vi "StateLED.vi"(0 "Master State":T1(ring)) -> ()   [LabVIEW 2019]
doc: "This VI manages the apperance of the LEDs. The LED coloration and blink pattern report the robot mode and status. See project documentation for details."
uses:
  outputs.vi
  dscommands.vi
  refnums.vi
  dsdata.vi
  sensors.vi
  autoninfo.vi
  <vilib>/vision/NI_Vision_Development_Module.lvlib
panel:
  in  "Shooter Firing":u32(colorbox)=61212
  in  "Shooter Ready":u32(colorbox)=16711758
  in  "User Value Choice":u8(slide)=255 step=1 scale=0.0..255.0
  in  "User Saturation Choice":u8(slide)=255 step=1 scale=0.0..255.0
  in  "Pressure Insert":u32(colorbox)=91
  in  "Battery Insert":u32(colorbox)=65282
  in  "Pressure Background":u32(colorbox)=16711680
  in  "Battery Background":u32(colorbox)=16711680
  in  "Pressure LED Length":i32=5
  in  "Battery LED Length":i32=5
  in  "Battery Index":i32=1
  in  "Pressure Index":i32=15
  in  "Swerve 3 LED Index":i32=20
  in  "Swerve 2 LED Index":i32
  in  "Swerve 1 LED Index":i32=6
  in  "Swerve LED Length":i32=1
  in  "Swerve 0 LED Index":i32=14
  in  "Locate LED":bool
  in  "LED Index":i32
  out "User Blue":u8
  out "User Green":u8=255
  out "User Red":u8
  in  "Choose Hue":bool
  in  "User Hue Choice":u8(slide) step=1 scale=0.0..255.0
  in  "Nominal Chase":u32(colorbox)=65280
  in  "Spinning":u32(colorbox)=16765440
  in  "Human Player Signal (blink)":u32(colorbox)=6618880
  in  "Diverting Power":u32(colorbox)
  in  "Master Caution Chase":u32(colorbox)=16711680
  in  "Autonomous Chase":u32(colorbox)=16727040
  in  "Human Driving":u32(colorbox)=43263
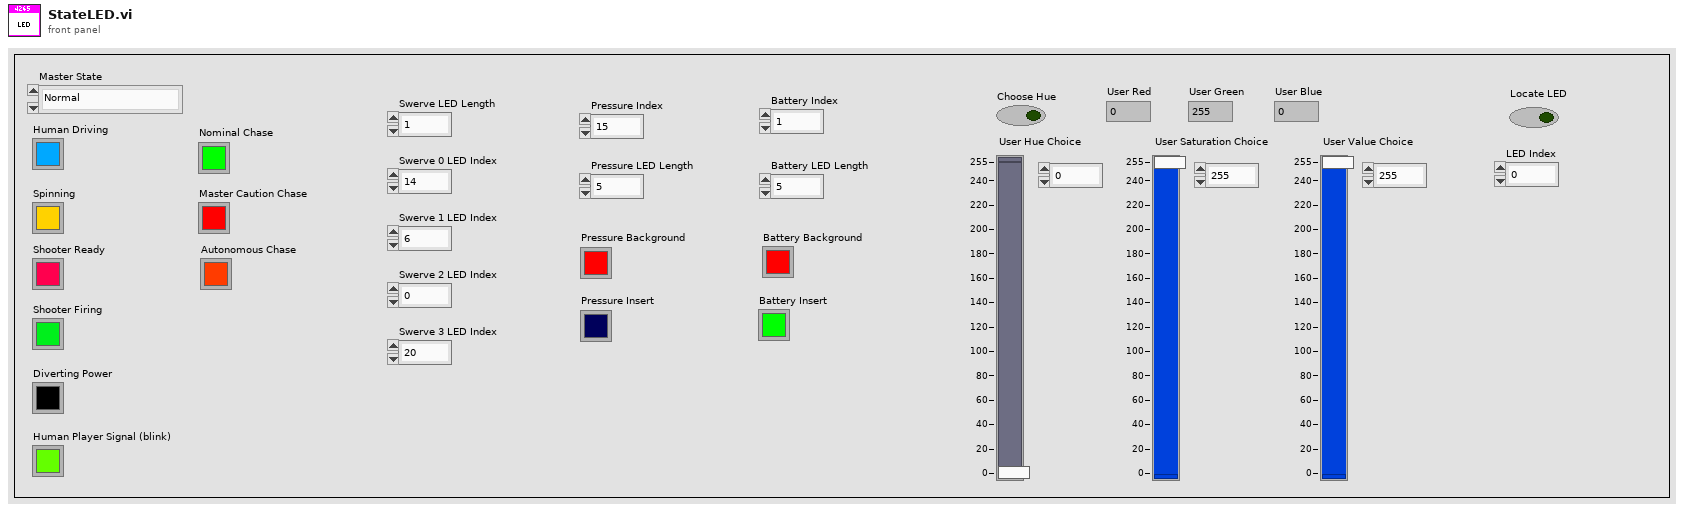
[diagram p1: front panel]
types:
  T1 = enum16{"Normal", "Control Rotation", "Control Position", "Climb"}
  T2 = enum16{"Normal", "Party Mode", "Choose Hue", "Debug", "Locate LED", "Rainbow Distance"}
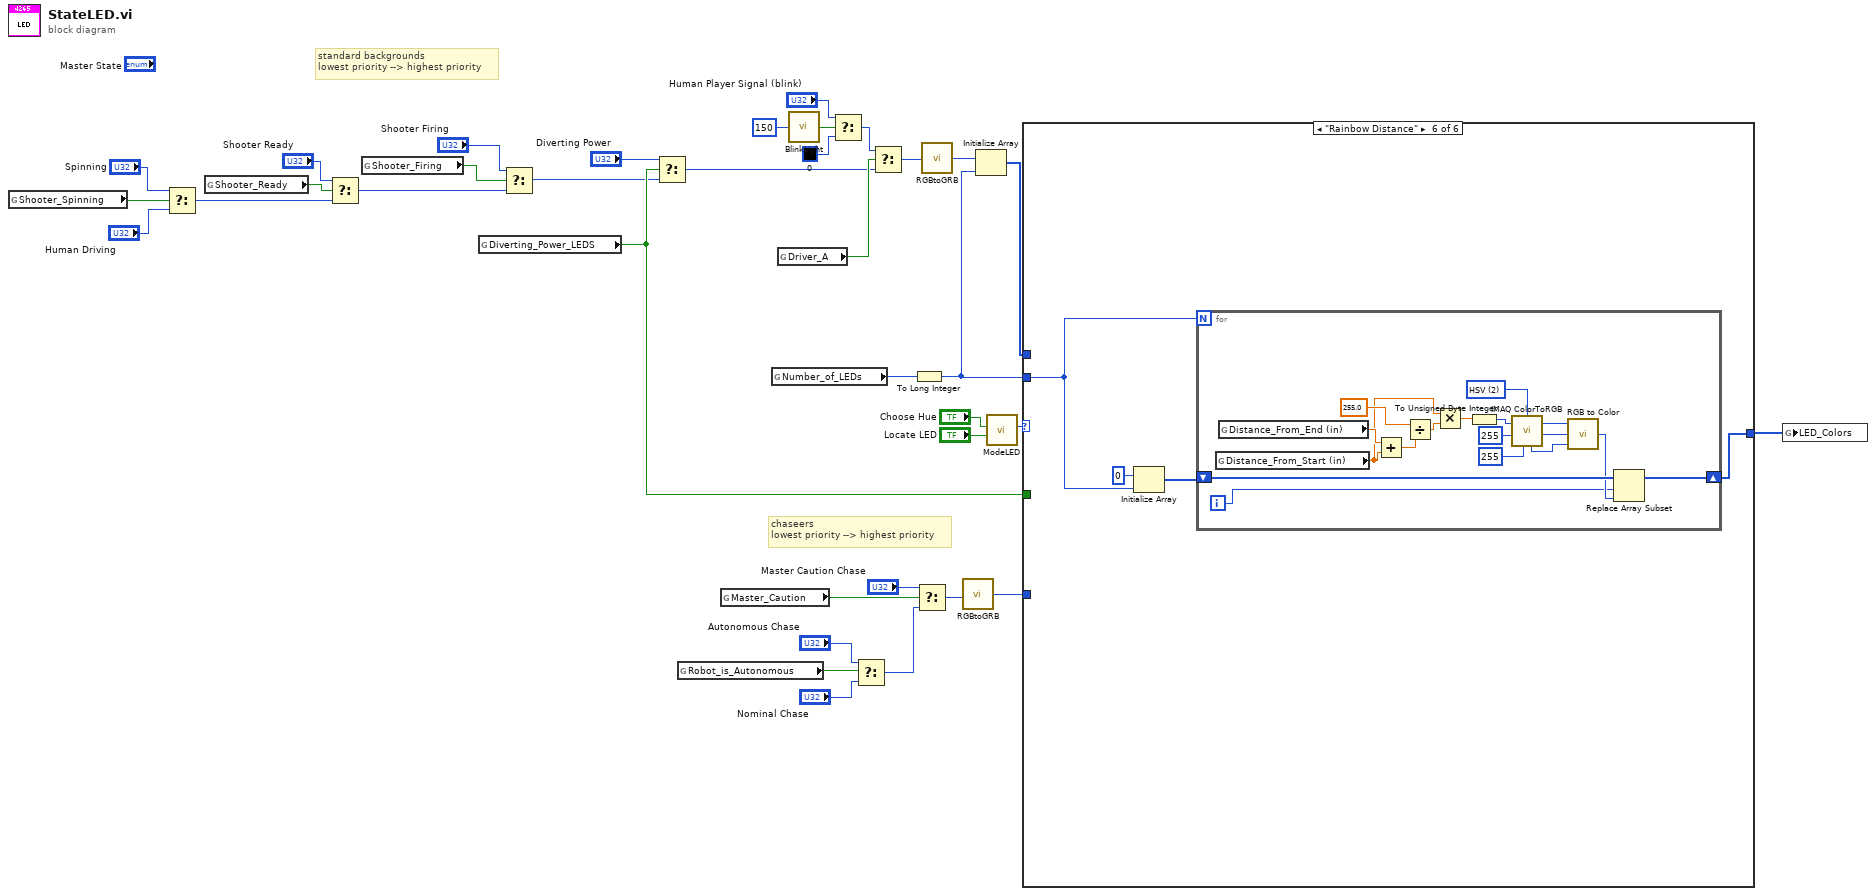
[diagram p0: block diagram]
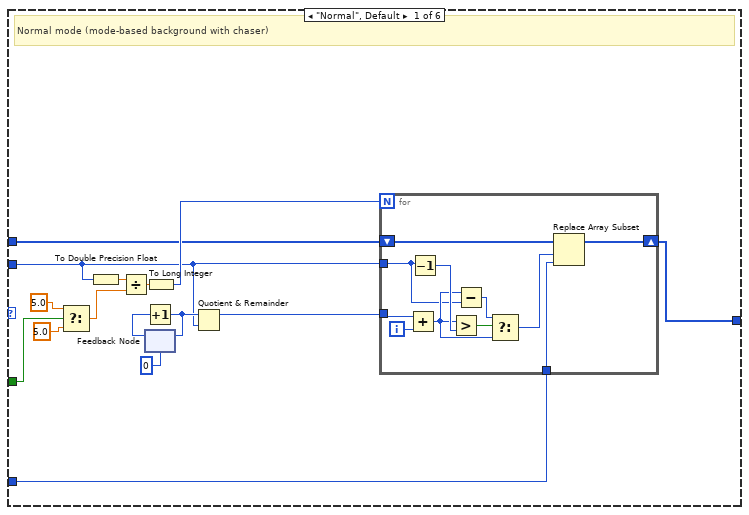
[diagram p2: hidden frame]
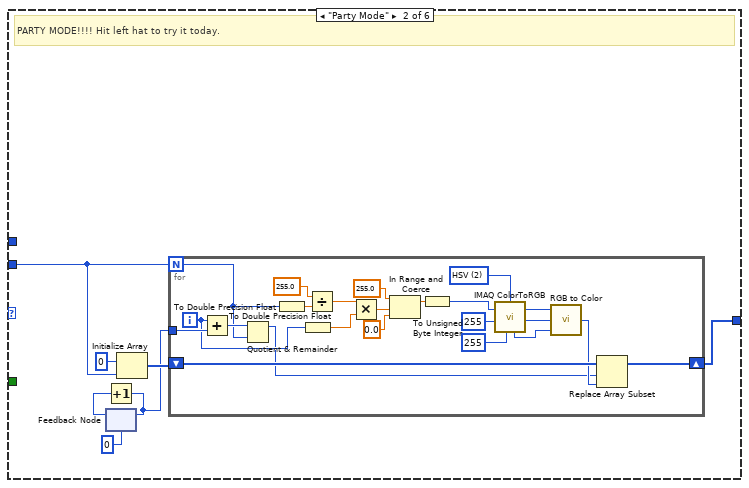
[diagram p3: hidden frame]
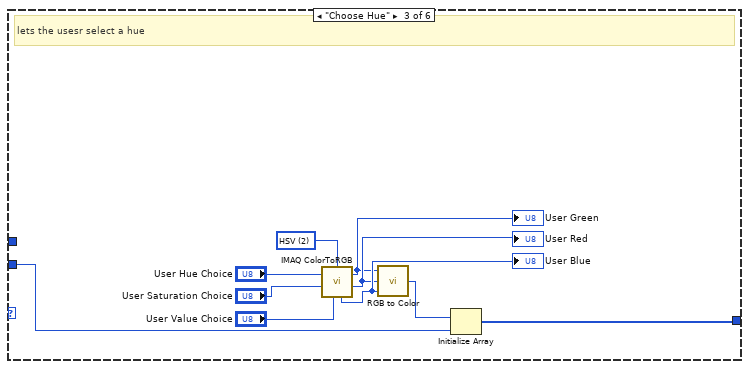
[diagram p4: hidden frame]
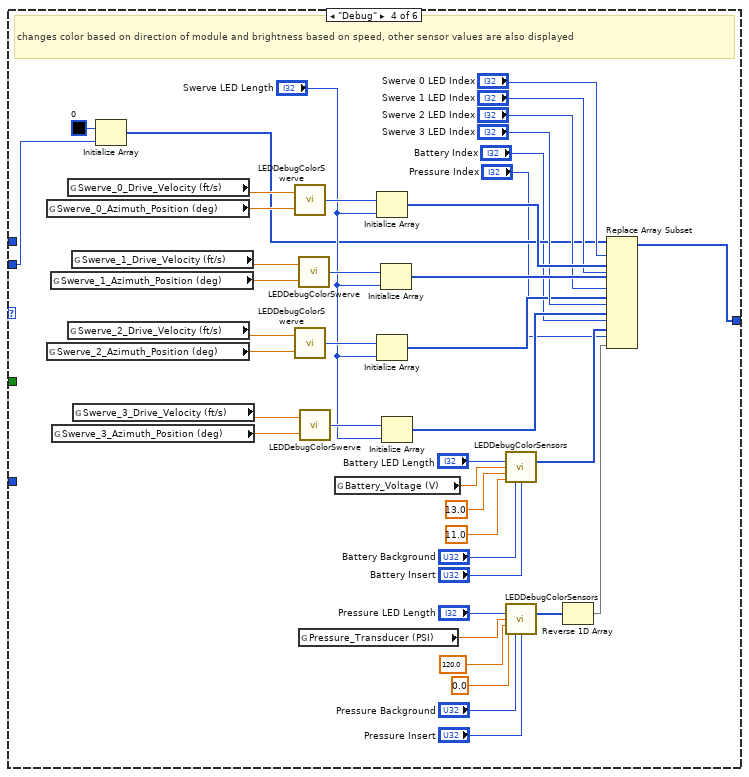
[diagram p5: hidden frame]
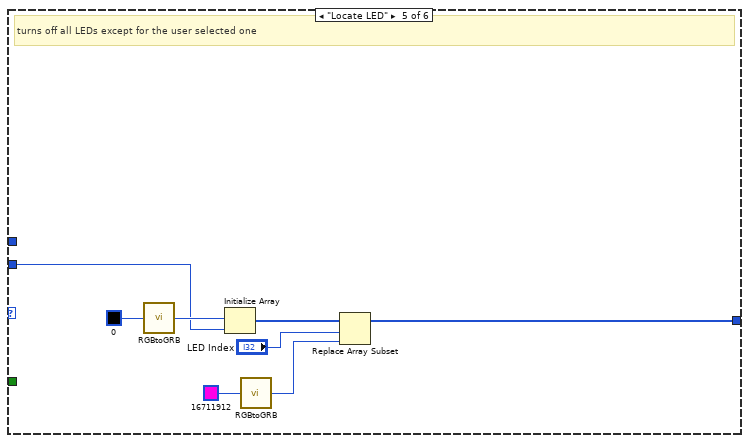
[diagram p6: hidden frame]
diagram:
  # "chaseers\nlowest priority --> highest priority"
  # "standard backgrounds\nlowest priority --> highest priority"
  n1 = global read "outputs.vi" "Shooter_Spinning"() -> (w12:bool)
  n2 = Select(t="Spinning", s=w12, f="Human Driving") -> (s? t:f=w36:u32)
  n3 = global read "outputs.vi" "Shooter_Ready"() -> (w9:bool)
  n4 = Select(t="Shooter Ready", s=w9, f=w36) -> (s? t:f=w8:u32)
  n5 = global read "outputs.vi" "Shooter_Firing"() -> (w7:bool)
  n6 = global read "outputs.vi" "Diverting_Power_LEDS"() -> (w14:bool)
  n7 = Select(t="Shooter Firing", s=w7, f=w8) -> (s? t:f=w6:u32)
  n8 = Select(t="Diverting Power", s=w14, f=w6) -> (s? t:f=w28:u32)
  n9 = global read "dsdata.vi" "Robot_is_Autonomous"() -> (w4:bool)
  n10 = global read "dsdata.vi" "Master_Caution"() -> (w23:bool)
  n11 = global read "refnums.vi" "Number_of_LEDs"() -> (w33:u16)
  n12 = global read "dscommands.vi" "Driver_A"() -> (w34:bool)
  n13 = call "BlinkLight.vi"("Blink Interval (ms)"=u32 150) -> ("Blinked Output"=w32:bool)
  n14 = Select(t="Human Player Signal (blink)", s=w32, f=u32 0 ("Color (RGB)")) -> (s? t:f=w29:u32)
  n15 = Select(t="Autonomous Chase", s=w4, f="Nominal Chase") -> (s? t:f=w1:u32)
  n16 = Select(t=w29, s=w34, f=w28) -> (s? t:f=w27:u32)
  n17 = To Long Integer(number=w33) -> (32bit integer=w16:i32)
  n18 = Select(t="Master Caution Chase", s=w23, f=w1) -> (s? t:f=w15:u32)
  n19 = call "RGBtoGRB.vi"("Color (RGB)"=w27) -> ("Color (GRB)"=w26:u32)
  n20 = call "RGBtoGRB.vi"("Color (RGB)"=w15) -> ("Color (GRB)"=w20:u32)
  n21 = Initialize Array(w26, w16) -> (w21:u32[])
  n22 = call "ModeLED.vi"("Locate LED"="Locate LED", "Choose Hue"="Choose Hue") -> ("LED Mode"=w19:T2)  [unwired: 9 in]
  n23 = case shown="\"Rainbow Distance\"" w19 {
    tunnel: w21 -> [w42 _ _ _ _ _]
    tunnel: [w41 w67 w96 w139 w146 w153] -> w22
    tunnel: w20 -> [w51 _ _ _ _ _]
    tunnel: w16 -> [w43 w64 w95 w122 w145 w154]
    tunnel: w14 -> [w38 _ _ _ _ _]
    frame "Normal", Default {
      # "Normal mode (mode-based background with chaser)"
      n24 = Select(t=5.0, s=w38, f=5.0 ("y")) -> (s? t:f=w39:dbl)
      n25 = To Double Precision Float(number=w43) -> (double precision float=w50:dbl)
      n26 = Divide(x=w50, y=w39) -> (x/y=w49:dbl)
      n27 = feedback #1(0) -> (w47:i32)
      n28 = Increment(x=w47) -> (x+1=w48:i32)
      n29 = feedback-in #1(w48) -> ()
      n30 = To Long Integer(number=w49) -> (32bit integer=w45:i32)
      n31 = Quotient & Remainder(x=w48, y=w43) -> (x-y*floor(x/y)=w44:i32)  [unwired: 1 out]
      n32 = for {
        N: w45 -> [_]
        tunnel: w44 -> [w62]
        tunnel: w43 -> [w53]
        shift-right: [w56] -> w41
        shift-left: w42 -> [w57]
        tunnel: w51 -> [w55]
        i -> [w59]
        n33 = Add(x=w62, y=w59) -> (x+y=w54:i32)
        n34 = Decrement(x=w53) -> (x-1=w61:i32)
        n35 = Greater?(x=w54, y=w61) -> (0:w60:bool)
        n36 = Subtract(x=w54, y=w53) -> (x-y=w52:i32)
        n37 = Select(t=w52, s=w60, f=w54) -> (s? t:f=w58:i32)
        n38 = Replace Array Subset(array=w57, new element=w55, index=w58) -> (w56:u32[])
      }
    }
    frame "Party Mode" {
      # "PARTY MODE!!!! Hit left hat to try it today."
      n39 = feedback #2(0) -> (w66:i32)
      n40 = Increment(x=w66) -> (x+1=w63:i32)
      n41 = feedback-in #2(w63) -> ()
      n42 = Initialize Array(u32 0 ("element"), w64) -> (w68:u32[])
      n43 = for {
        N: w64 -> [w72]
        shift-right: [w80] -> w67
        shift-left: w68 -> [w81]
        tunnel: w63 -> [w74]
        i -> [w71]
        w90 = u16 2 items=["RGB", "HSL", "HSV", "HSI"] ("Color Mode")
        n44 = Add(x=w71, y=w74) -> (x+y=w73:i32)
        n45 = Quotient & Remainder(x=w73, y=w72) -> (x-y*floor(x/y)=w70:i32)  [unwired: 1 out]
        n46 = To Double Precision Float(number=w72) -> (double precision float=w89:dbl)
        n47 = To Double Precision Float(number=w71) -> (double precision float=w86:dbl)
        n48 = Divide(x=255.0, y=w89) -> (x/y=w87:dbl)
        n49 = Multiply(x=w87, y=w86) -> (x*y=w85:dbl)
        n50 = In Range and Coerce(upper limit=255.0, x=w85, lower limit=0.0) -> (coerced(x)=w82:dbl)  [unwired: 1 out]
        n51 = To Unsigned Byte Integer(number=w82) -> (unsigned 8bit integer=w75:u8)
        n52 = call "IMAQ ColorToRGB"("Green or Sat value"=u8 255, "Blue or Luma or Val or Inten value"=u8 255, "Red or Hue value"=w75, "Color Mode"=w90) -> ("Blue value"=w76:u8, "Green value"=w77:u8, "Red value"=w78:u8)  [unwired: 1 in, 1 out]
        n53 = call <vilib>:"RGB to Color.vi"("B"=w76, "G"=w77, "R"=w78) -> ("Color"=w79:u32)
        n54 = Replace Array Subset(array=w81, new element=w79, index=w70) -> (w80:u32[])
      }
    }
    frame "Choose Hue" {
      w98 = u16 2 items=["RGB", "HSL", "HSV", "HSI"] ("Color Mode")
      # "lets the usesr select a hue"
      n55 = call "IMAQ ColorToRGB"("Green or Sat value"="User Saturation Choice", "Blue or Luma or Val or Inten value"="User Value Choice", "Red or Hue value"="User Hue Choice", "Color Mode"=w98) -> ("Blue value"=w101:u8, "Green value"=w100:u8, "Red value"=w99:u8)  [unwired: 1 in, 1 out]
      "User Red" <- w100
      "User Green" <- w99
      "User Blue" <- w101
      n56 = call <vilib>:"RGB to Color.vi"("B"=w101, "G"=w100, "R"=w99) -> ("Color"=w97:u32)
      n57 = Initialize Array(w97, w95) -> (w96:u32[])
    }
    frame "Debug" {
      # "changes color based on direction of module and brightness based on speed, other sensor values are also displayed"
      n58 = global read "sensors.vi" "Swerve_0_Azimuth_Position (deg)"() -> (w143:dbl)
      n59 = global read "sensors.vi" "Swerve_2_Azimuth_Position (deg)"() -> (w126:dbl)
      n60 = global read "sensors.vi" "Swerve_1_Azimuth_Position (deg)"() -> (w136:dbl)
      n61 = global read "sensors.vi" "Swerve_3_Azimuth_Position (deg)"() -> (w129:dbl)
      n62 = global read "sensors.vi" "Swerve_0_Drive_Velocity (ft/s)"() -> (w144:dbl)
      n63 = global read "sensors.vi" "Swerve_2_Drive_Velocity (ft/s)"() -> (w128:dbl)
      n64 = global read "sensors.vi" "Swerve_1_Drive_Velocity (ft/s)"() -> (w138:dbl)
      n65 = global read "sensors.vi" "Swerve_3_Drive_Velocity (ft/s)"() -> (w131:dbl)
      n66 = Initialize Array(u32 0 ("Color (RGB)"), w122) -> (w120:u32[])
      n67 = call "LEDDebugColorSwerve.vi"("Azimuth_Angle (deg [-180,180])"=w143, "Drive Velocity (ft/s)"=w144) -> ("Color"=w141:u32)
      n68 = call "LEDDebugColorSwerve.vi"("Azimuth_Angle (deg [-180,180])"=w126, "Drive Velocity (ft/s)"=w128) -> ("Color"=w127:u32)
      n69 = call "LEDDebugColorSwerve.vi"("Azimuth_Angle (deg [-180,180])"=w136, "Drive Velocity (ft/s)"=w138) -> ("Color"=w137:u32)
      n70 = global read "sensors.vi" "Pressure_Transducer (PSI)"() -> (w107:dbl)
      n71 = call "LEDDebugColorSwerve.vi"("Azimuth_Angle (deg [-180,180])"=w129, "Drive Velocity (ft/s)"=w131) -> ("Color"=w130:u32)
      n72 = global read "sensors.vi" "Battery_Voltage (V)"() -> (w119:dbl)
      n73 = Initialize Array(w141, "Swerve LED Length") -> (w140:u32[])
      n74 = Initialize Array(w127, "Swerve LED Length") -> (w124:u32[])
      n75 = Initialize Array(w137, "Swerve LED Length") -> (w135:u32[])
      n76 = Initialize Array(w130, "Swerve LED Length") -> (w123:u32[])
      n77 = call "LEDDebugColorSensors.vi"("LED Length"="Battery LED Length", "Value"=w119, "Max"=13.0, "Min"=11.0, "Background Color"="Battery Background", "Color to Insert"="Battery Insert") -> ("Output Color Array"=w116:u32[])  [unwired: 9 in]
      n78 = call "LEDDebugColorSensors.vi"("LED Length"="Pressure LED Length", "Value"=w107, "Max"=120.0, "Min"=0.0, "Background Color"="Pressure Background", "Color to Insert"="Pressure Insert") -> ("Output Color Array"=w104:u32[])  [unwired: 9 in]
      n79 = Reverse 1D Array(array=w104) -> (reversed array=w103:u32[])
      n80 = Replace Array Subset(array=w120, new element #1=w140, index #1="Swerve 0 LED Index", new element #2=w135, index #2="Swerve 1 LED Index", new element #3=w124, index #3="Swerve 2 LED Index", new element #4=w123, index #4="Swerve 3 LED Index", new element #5=w116, index #5="Battery Index", new element #6=w103, index #6="Pressure Index") -> (w139:u32[])
    }
    frame "Locate LED" {
      # "turns off all LEDs except for the user selected one"
      n81 = call "RGBtoGRB.vi"("Color (RGB)"=u32 0) -> ("Color (GRB)"=w151:u32)
      n82 = Initialize Array(w151, w145) -> (w150:u32[])
      n83 = call "RGBtoGRB.vi"("Color (RGB)"=u32 16711912) -> ("Color (GRB)"=w148:u32)
      n84 = Replace Array Subset(array=w150, new element=w148, index="LED Index") -> (w146:u32[])
    }
    frame "Rainbow Distance" {
      n85 = Initialize Array(u32 0 ("element"), w154) -> (w155:u32[])
      n86 = for {
        N: w154 -> [_]
        shift-right: [w169] -> w153
        shift-left: w155 -> [w170]
        i -> [w157]
        w171 = u16 2 items=["RGB", "HSL", "HSV", "HSI"] ("Color Mode")
        n87 = global read "autoninfo.vi" "Distance_From_Start (in)"() -> (w160:dbl)
        n88 = global read "autoninfo.vi" "Distance_From_End (in)"() -> (w164:dbl)
        n89 = Add(x=w164, y=w160) -> (x+y=w163:dbl)
        n90 = Divide(x=255.0, y=w163) -> (x/y=w161:dbl)
        n91 = Multiply(x=w160, y=w161) -> (x*y=w158:dbl)
        n92 = To Unsigned Byte Integer(number=w158) -> (unsigned 8bit integer=w159:u8)
        n93 = call "IMAQ ColorToRGB"("Green or Sat value"=u8 255, "Blue or Luma or Val or Inten value"=u8 255, "Red or Hue value"=w159, "Color Mode"=w171) -> ("Blue value"=w165:u8, "Green value"=w166:u8, "Red value"=w167:u8)  [unwired: 1 in, 1 out]
        n94 = call <vilib>:"RGB to Color.vi"("B"=w165, "G"=w166, "R"=w167) -> ("Color"=w168:u32)
        n95 = Replace Array Subset(array=w170, new element=w168, index=w157) -> (w169:u32[])
      }
    }
  }
  n96 = global write "outputs.vi" "LED_Colors"(w22) -> ()
